vi "fgv_Ntrip-Client_config.vi"(7 "cmd":T2, 11 "Ntrip client val":T1={"Ntrip client set-val"={"id"="seoul", "pwd"="seoul", "ref pt"="YONS-RTCM32-M5", "address"="gnss.eseoul.go.kr", "port "=2101}, "Mount points"=0} {"Mount points" items=["SONP-RTCM32", "GANS-RTCM32", "GUMC-RTCM32", "DBON-RTCM32", "YONS-RTCM23", "SONP-RTCM23", "GUMC-RTCM23", "GANS-RTCM31", "YONS-CMRx", "SONP-RTCM31", "GUMC-RTCM31", "GANS-RTCM23", "DBON-RTCM23", "DBON-RTCM31", "YONS-RTCM31", "YONS-RTCM32-M5", "VRS-RTCM32-M5", "VRS-RTCM31", "VRS-CMRx", "VRS-CMRplus"]}) -> (3 "Ntrip client val out":T1={"Ntrip client set-val"={"id"="seoul", "pwd"="seoul", "ref pt"="YONS-RTCM32-M5", "address"="gnss.eseoul.go.kr", "port "=2101}, "Mount points"=0} {"Mount points" items=["SONP-RTCM32", "GANS-RTCM32", "GUMC-RTCM32", "DBON-RTCM32", "YONS-RTCM23", "SONP-RTCM23", "GUMC-RTCM23", "GANS-RTCM31", "YONS-CMRx", "SONP-RTCM31", "GUMC-RTCM31", "GANS-RTCM23", "DBON-RTCM23", "DBON-RTCM31", "YONS-RTCM31", "YONS-RTCM32-M5", "VRS-RTCM32-M5", "VRS-RTCM31", "VRS-CMRx", "VRS-CMRplus"]})   [LabVIEW 2019]
uses:
  Ctrl/cmd_common.ctl
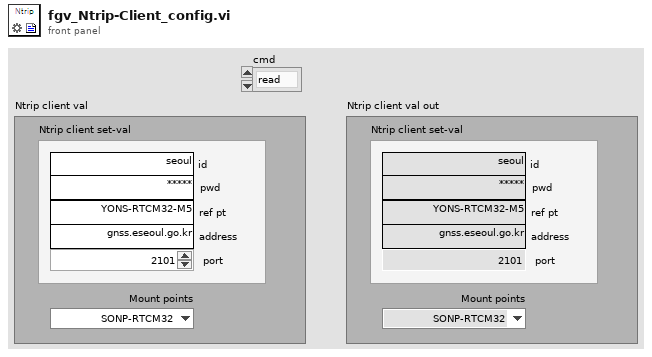
[diagram p1: front panel]
types:
  T1 = cluster{"Ntrip client set-val":cluster{"id":string, "pwd":string, "ref pt":string, "address":string, "port ":u16}, "Mount points":u16}
  T2 = typedef "cmd_common.ctl" = enum16{"read", "write"}
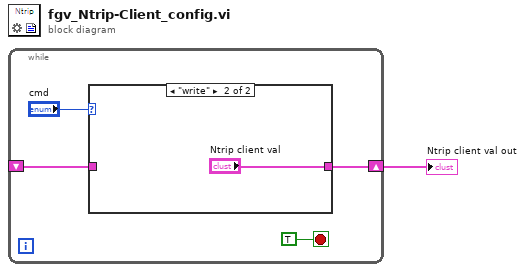
[diagram p0: block diagram]
diagram:
  n1 = while {
    shift-right: [w3] -> w1
    shift-left: _ -> [w2]
    stop <- TRUE stop-if-true
    n2 = case shown="\"write\"" "cmd" {
      tunnel: [w6 "Ntrip client val"] -> w3
      tunnel: w2 -> [w6 _]
      frame "read", Default {
      }
      frame "write" {
      }
    }
  }
  "Ntrip client val out" <- w1
